vi "OAT Sampled Power Spectrum (Multi Channels).vi"(6 "window info":T3={"window type"=10, "window length"=2048} {"window type" items=["None"=0, "Hanning"=1, "Hamming"=2, "Blackman-Harris"=3, "Exact Blackman"=4, "Blackman"=5, "Flat Top"=6, "4 Term B-Harris"=7, "7 Term B-Harris"=8, "Low Sidelobe"=9, "Gaussian"=62]; "window length" min=0}, 7 "dB On (T)":bool=TRUE, 8 "error in (no error)":errorcluster, 10 "channel info":T1(array[cluster]) {"pregain [dB]" format="%.2f"; "dB reference [EU]" format="%.1e"; "sensor sensitivity [mV/EU]" format="%.2f"}, 11 "resampled signals":cluster{"r0":dbl, "dr":dbl, "Y":dbl[]}[](array[cluster]) {"r0" format="%.2p"; "dr" format="%.2p"; "Y" format="%.2f"}) -> (0 "error out":errorcluster, 2 "unit label":string[](array[string]), 3 "order spectrums":T2(array[cluster]) {"order 0" format="%.2p"; "delta order" format="%.2p"; "magnitude" format="%.2f"})   [LabVIEW 2017]
doc: "Computes the single-sided, scaled auto power spectrums of time-domain signals sampled from multiple channels. You can define the number of frequency bins."
uses:
  <vilib>/addons/Sound and Vibration/Order Analysis/Ref Gabor Order Tracking/window information.ctl
  <vilib>/addons/Sound and Vibration/Order Analysis/Resample Order Tracking/SubVIs/OAT Verify Resampled Signal (Multi Channels).vi
  <vilib>/Analysis/NI_AALPro.lvlib
  <vilib>/addons/Sound and Vibration/Order Analysis/Resample Order Tracking/SoundVib_Resampling.lvlib
  <vilib>/addons/Sound and Vibration/Order Analysis/Gabor Order Tracking/SoundVib_Gabor.lvlib
panel:
  # "OAT Sampled Power Spectrum (Multi Channels)"
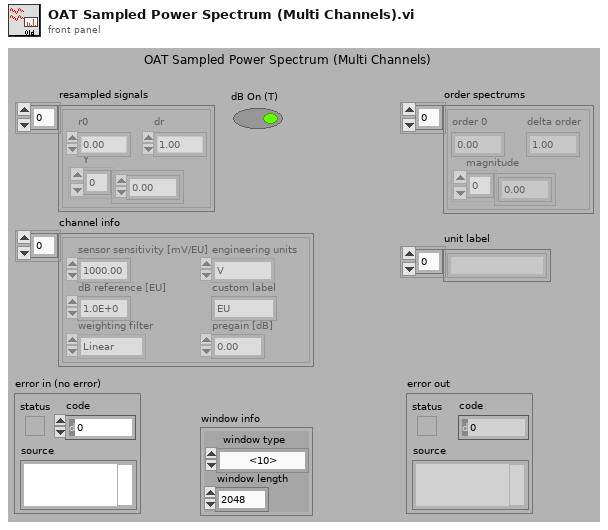
[diagram p1: front panel]
types:
  T1 = cluster{"sensor sensitivity [mV/EU]":dbl, "engineering units":enum16{"custom...", "V", "Pa", "g", "m/s^2", "m/s", "m", "in/s^2", "in/s", "in"}, "dB reference [EU]":dbl, "custom label":string, "weighting filter":enum16{"Linear", "A-weighting", "B-weighting", "C-weighting"}, "pregain [dB]":dbl}[]
  T2 = cluster{"order 0":dbl, "delta order":dbl, "magnitude":dbl[]}[]
  T3 = typedef "SoundVib_Gabor.lvlib/window information.ctl" = cluster{"window type":u32, "window length":i32}
  T4 = cluster{"df":dbl, "df":dbl, "log view [dB EU]":dbl[]}[]
  T5 = cluster{"sensor sensitivity [mV/EU]":dbl, "engineering units":enum16{"custom...", "V", "Pa", "g", "m/s^2", "m/s", "m", "in/s^2", "in/s", "in"}, "dB reference [EU]":dbl, "custom label":string, "weighting filter":enum16{"Linear", "A-weighting", "B-weighting", "C-weighting"}, "pregain [dB]":dbl}
  T6 = cluster{"df":dbl, "df":dbl, "log view scaled signal":dbl[]}
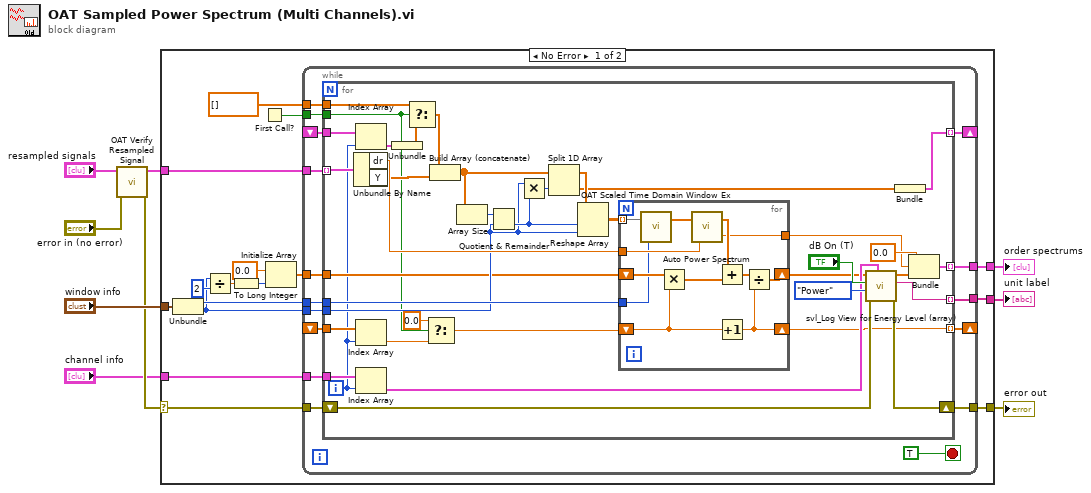
[diagram p0: block diagram]
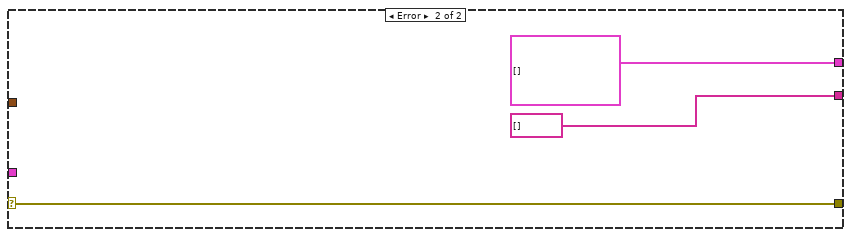
[diagram p2: hidden frame]
diagram:
  n1 = call-poly <vilib>:"OAT Verify Resampled Signal.vi"("error in (no error)"="error in (no error)", "resampled signal"="resampled signals") -> ("error out"=w8:errorcluster, "resampled signal out"=w1:cluster{"r0":dbl, "dr":dbl, "Y":dbl[]}[])  [unwired: 7 in, 1 out]
  n2 = case shown="No Error" w8 {
    selector: w8 -> [w21 w94]
    tunnel: "window info" -> [w15 _]
    tunnel: [w25 string[] []] -> w2
    tunnel: [w24 T4 []] -> w4
    tunnel: "channel info" -> [w23 _]
    tunnel: [w20 w94] -> w6
    tunnel: w1 -> [w22 _]
    frame No Error {
      n3 = Unbundle(w15) -> ("window type"=w14:u32, "window length"=w13:i32)
      n4 = Divide(x=w13, y=2) -> (x/y=w17:dbl)
      n5 = To Long Integer(number=w17) -> (32bit integer=w19:i32)
      n6 = First Call?() -> (First Call?: T/F=w12:bool)
      n7 = Initialize Array(0.0 ("Element Data"), w19) -> (w10:dbl[])
      n8 = while {
        tunnel: [w41] -> w25
        tunnel: [w40] -> w24
        tunnel: w23 -> [w39]
        tunnel: w22 -> [w38]
        tunnel: w21 -> [w37]
        tunnel: [w36] -> w20
        tunnel: w14 -> [w35]
        tunnel: w13 -> [w34]
        shift-right: [w33] -> _
        shift-left: _ -> [w32]
        tunnel: w12 -> [w30]
        tunnel: dbl[] [] -> [w29]
        tunnel: w10 -> [w28]
        shift-right: [w27] -> _
        shift-left: _ -> [w26]
        stop <- TRUE stop-if-true
        n9 = for {
          tunnel: [w76] -> w41 mode=indexing
          tunnel: [w73] -> w40 mode=indexing
          tunnel: w39 -> [w67]
          tunnel: w38 -> [w72] mode=indexing
          shift-right: [w70] -> w36
          shift-left: w37 -> [w71]
          tunnel: w35 -> [w65]
          tunnel: w34 -> [w59]
          tunnel: [w61] -> w33 mode=indexing
          tunnel: w32 -> [w57]
          tunnel: w30 -> [w49]
          tunnel: w29 -> [w54]
          tunnel: w28 -> [w50]
          tunnel: [w46] -> w27 mode=indexing
          tunnel: w26 -> [w45]
          i -> [w44]
          n10 = Unbundle By Name(w72) -> ("dr"=w69:dbl, "Y"=w53:dbl[])
          n11 = Index Array(array=w57, index=w44) -> (element=w56:cluster{dbl[]})
          n12 = Index Array(array=w45, index=w44) -> (element=w43:dbl)
          n13 = Index Array(array=w67, index=w44) -> (element=w66:T5)
          n14 = Unbundle(w56) -> (w55:dbl[])
          n15 = Select(t=w54, s=w49, f=w55) -> (s? t:f=w51:dbl[])
          n16 = Select(t=0.0, s=w49, f=w43) -> (s? t:f=w47:dbl)
          n17 = Build Array (concatenate)(w51, w53) -> (w52:dbl[])
          n18 = Array Size(array=w52) -> (size(s)=w79:i32)
          n19 = Quotient & Remainder(x=w79, y=w59) -> (floor(x/y)=w60:i32)  [unwired: 1 out]
          n20 = Multiply(x=w59, y=w60) -> (x*y=w58:i32)
          n21 = Split 1D Array(array=w52, index=w58) -> (first subarray=w63:dbl[], second subarray=w62:dbl[])
          n22 = Reshape Array(w63, w60, w59) -> (w64:dbl[][])
          n23 = for {
            tunnel: w64 -> [w87] mode=indexing
            shift-right: [w81] -> w42
            shift-left: w50 -> [w91]
            tunnel: w69 -> [w89]
            tunnel: [w88] -> w68
            tunnel: w65 -> [w85]
            shift-right: [w80] -> w46
            shift-left: w47 -> [w83]
            n24 = call <vilib>:"OAT Scaled Time Domain Window Ex.vi"("window type"=w85, "X"=w87) -> ("y"=w86:dbl[])  [unwired: 1 out]
            n25 = Multiply(x=w91, y=w83) -> (x*y=w84:dbl[])
            n26 = call <vilib>:"Auto Power Spectrum.vi"("dt"=w89, "Signal (V)"=w86) -> ("df"=w88:dbl, "Power Spectrum (V^2 rms)"=w90:dbl[])
            n27 = Add(x=w90, y=w84) -> (x+y=w82:dbl[])
            n28 = Increment(x=w83) -> (x+1=w80:dbl)
            n29 = Divide(x=w82, y=w80) -> (x/y=w81:dbl[])
          }
          n30 = call <vilib>:"svl_Log View for Energy Level (array).vi"("channel info"=w66, "error in (no error)"=w71, "view mode"=enum16{"Power", "Amplitude"}."Power", "dB On (T)"="dB On (T)", "scaled signal"=w42) -> ("error out"=w70:errorcluster, "unit label"=w76:string, "log view scaled signal"=w75:dbl[])  [unwired: 4 in]
          n31 = Bundle(w62) -> (w61:cluster{dbl[]})  [unwired: 1 in]
          n32 = Bundle("df"=0.0, "df"=w68, "log view scaled signal"=w75) -> (w73:T6)  [unwired: 1 in]
        }
      }
    }
    frame Error {
    }
  }
  "error out" <- w6
  "order spectrums" <- w4
  "unit label" <- w2
